vi "DIO-ApplyCorrection.vi"(2 "TaskCluster":T2, 7 "NordSud(ms)":i32, 11 "EstOuest(ms)":i32, 13 "ReferenceCluster":T1) -> (8 "GuiderRA Error":errorcluster, 15 "GuiderDEC Error":errorcluster)   [LabVIEW 2019]
uses:
  <vilib>/DAQmx/write.llb/DAQmx Write (Digital Bool 1Line 1Point).vi
  <vilib>/DAQmx/miscellaneous.llb/DAQmx Fill In Error Info.vi
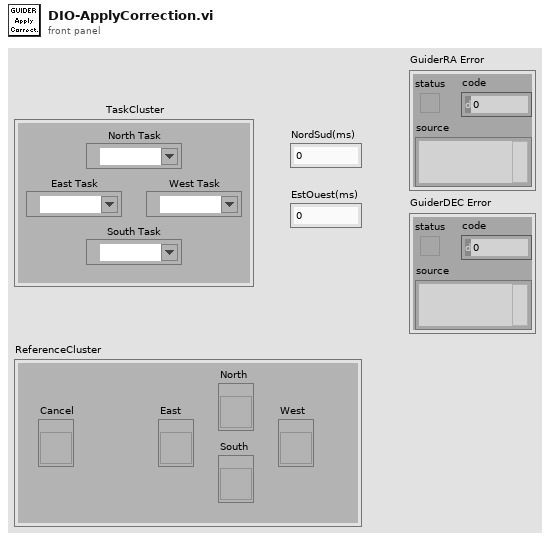
[diagram p1: front panel]
types:
  T1 = cluster{"Cancel":refnum<vi>, "North":refnum<vi>, "South":refnum<vi>, "East":refnum<vi>, "West":refnum<vi>}
  T2 = cluster{"North Task":refnum<k21>, "South Task":refnum<k21>, "East Task":refnum<k21>, "West Task":refnum<k21>}
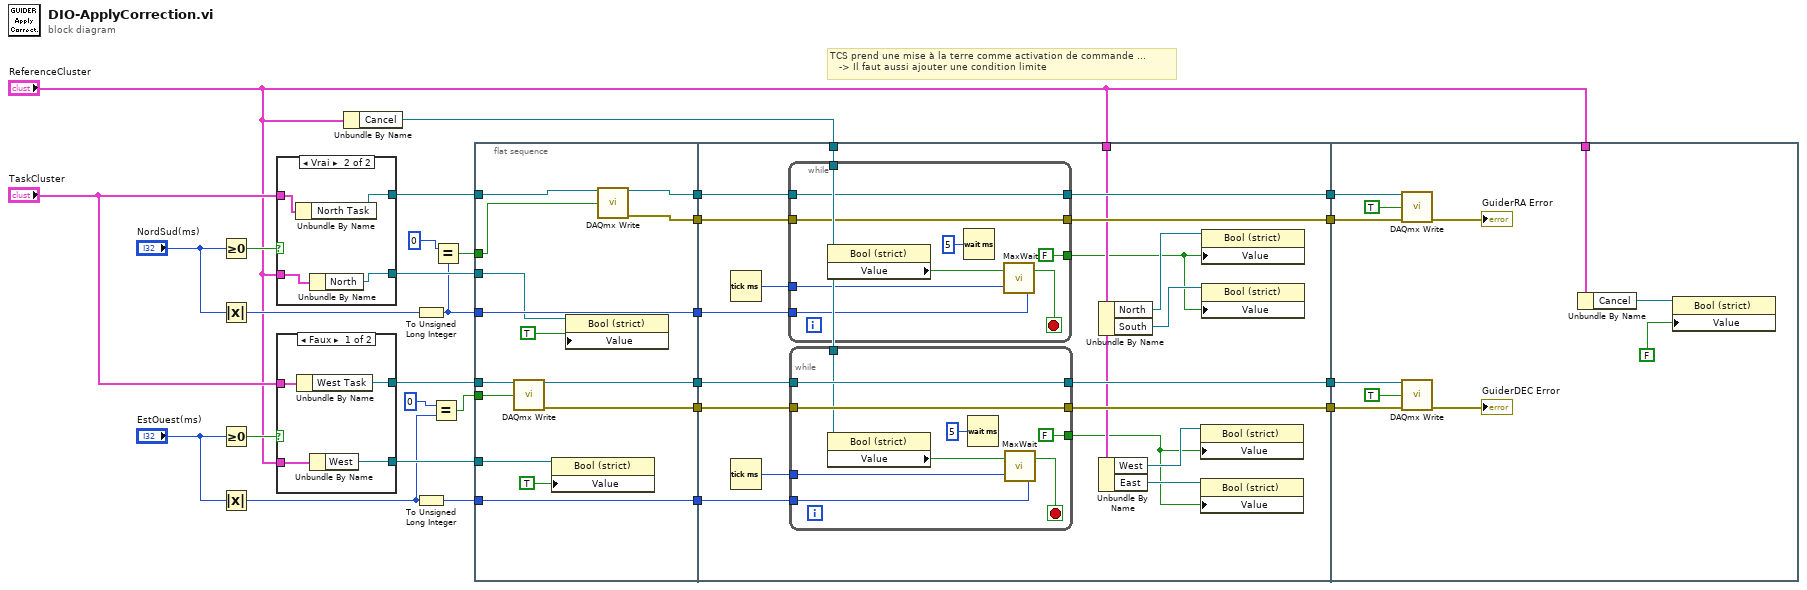
[diagram p0: block diagram]
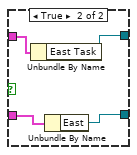
[diagram p2: hidden frame]
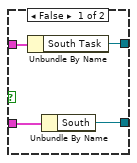
[diagram p3: hidden frame]
diagram:
  # "TCS prend une mise à la terre comme activation de commande ...\n   -> Il faut aussi ajouter une condition limite"
  n1 = Greater Or Equal To 0?(x="NordSud(ms)") -> (x >= 0?=w29:bool)
  n2 = Absolute Value(x="NordSud(ms)") -> (abs(x)=w24:i32)
  n3 = Greater Or Equal To 0?(x="EstOuest(ms)") -> (x >= 0?=w27:bool)
  n4 = Absolute Value(x="EstOuest(ms)") -> (abs(x)=w3:i32)
  n5 = case shown="Vrai" w29 {
    tunnel: "TaskCluster" -> [w33 w37]
    tunnel: [w32 w36] -> w12
    tunnel: "ReferenceCluster" -> [w31 w35]
    tunnel: [w30 w34] -> w15
    frame False {
      n6 = Unbundle By Name(w33) -> ("South Task"=w32:refnum<k21>)
      n7 = Unbundle By Name(w31) -> ("South"=w30:refnum<vi>)
    }
    frame True {
      n8 = Unbundle By Name(w37) -> ("North Task"=w36:refnum<k21>)
      n9 = Unbundle By Name(w35) -> ("North"=w34:refnum<vi>)
    }
  }
  n10 = case shown="Faux" w27 {
    tunnel: "TaskCluster" -> [w41 w45]
    tunnel: [w40 w44] -> w13
    tunnel: "ReferenceCluster" -> [w39 w43]
    tunnel: [w38 w42] -> w14
    frame False {
      n11 = Unbundle By Name(w41) -> ("West Task"=w40:refnum<k21>)
      n12 = Unbundle By Name(w39) -> ("West"=w38:refnum<vi>)
    }
    frame True {
      n13 = Unbundle By Name(w45) -> ("East Task"=w44:refnum<k21>)
      n14 = Unbundle By Name(w43) -> ("East"=w42:refnum<vi>)
    }
  }
  n15 = Unbundle By Name("ReferenceCluster") -> ("Cancel"=w16:refnum<vi>)
  n16 = To Unsigned Long Integer(number=w24) -> (unsigned 32bit integer=w6:u32)
  n17 = To Unsigned Long Integer(number=w3) -> (unsigned 32bit integer=w23:u32)
  n18 = Equal?(x=0, y=w3) -> (x = y?=w1:bool)
  n19 = Equal?(x=u32 0, y=w6) -> (x = y?=w4:bool)
  n20 = flat-sequence {
    tunnel: w23 -> [w58]
    tunnel: w13 -> [w57]
    tunnel: w12 -> [w54]
    tunnel: w6 -> [w59]
    tunnel: [w59] -> w22
    tunnel: [w53] -> w21
    tunnel: [w52] -> w20
    tunnel: [w56] -> w19
    tunnel: [w55] -> w18
    tunnel: [w58] -> w17
    tunnel: w15 -> [w51]
    tunnel: w14 -> [w50]
    tunnel: w4 -> [w47]
    tunnel: w1 -> [w46]
    tunnel: w16 -> [w67]
    tunnel: w22 -> [w79]
    tunnel: w21 -> [w78]
    tunnel: w20 -> [w75]
    tunnel: w19 -> [w73]
    tunnel: w18 -> [w72]
    tunnel: w17 -> [w69]
    tunnel: [w77] -> w11
    tunnel: [w76] -> w10
    tunnel: [w71] -> w9
    tunnel: [w70] -> w8
    tunnel: "ReferenceCluster" -> [w66]
    tunnel: w11 -> [w104]
    tunnel: w10 -> [w103]
    tunnel: w9 -> [w102]
    tunnel: w8 -> [w101]
    tunnel: "ReferenceCluster" -> [w100]
    frame #0 {
      n21 = call-poly <vilib>:"DAQmx Write.vi"("task/channels in"=w57, "data"=w46) -> ("task out"=w56:refnum<k21>, "error out"=w55:errorcluster)  [unwired: 11 in, 1 out]
      n22 = property class="Bool (strict)"(reference=w50, "Value"=TRUE) -> ()  [unwired: 1 in, 2 out]
      n23 = property class="Bool (strict)"(reference=w51, "Value"=TRUE) -> ()  [unwired: 1 in, 2 out]
      n24 = call-poly <vilib>:"DAQmx Write.vi"("task/channels in"=w54, "data"=w47) -> ("task out"=w53:refnum<k21>, "error out"=w52:errorcluster)  [unwired: 11 in, 1 out]
    }
    frame #1 {
      n25 = Tick Count (ms)() -> (millisecond timer value=w74:u32)
      n26 = Tick Count (ms)() -> (millisecond timer value=w68:u32)
      n27 = while {
        tunnel: w79 -> [w94]
        tunnel: w78 -> [w97]
        tunnel: [w97] -> w77
        tunnel: w75 -> [w96]
        tunnel: [w96] -> w76
        tunnel: w74 -> [w95]
        tunnel: w67 -> [w91]
        tunnel: [FALSE] -> w63
        stop <- w93 stop-if-true
        n28 = property class="Bool (strict)"(reference=w91) -> ("Value"=w92:bool)  [unwired: 1 in, 2 out]
        n29 = Wait (ms)(milliseconds to wait=u32 5) -> ()  [unwired: 1 out]
        n30 = call "MaxWait.vi"("WaitLimit (ms)"=w94, "StartTick (from outside the node)"=w95, "Valeur entrante"=w92) -> ("break ?"=w93:bool)
      }
      n31 = while {
        tunnel: w69 -> [w85]
        tunnel: w73 -> [w88]
        tunnel: [w88] -> w71
        tunnel: w72 -> [w87]
        tunnel: [w87] -> w70
        tunnel: w68 -> [w86]
        tunnel: w67 -> [w82]
        tunnel: [FALSE] -> w60
        stop <- w84 stop-if-true
        n32 = property class="Bool (strict)"(reference=w82) -> ("Value"=w83:bool)  [unwired: 1 in, 2 out]
        n33 = Wait (ms)(milliseconds to wait=u32 5) -> ()  [unwired: 1 out]
        n34 = call "MaxWait.vi"("WaitLimit (ms)"=w85, "StartTick (from outside the node)"=w86, "Valeur entrante"=w83) -> ("break ?"=w84:bool)
      }
      n35 = Unbundle By Name(w66) -> ("North"=w65:refnum<vi>, "South"=w64:refnum<vi>)
      n36 = Unbundle By Name(w66) -> ("West"=w61:refnum<vi>, "East"=w62:refnum<vi>)
      n37 = property class="Bool (strict)"(reference=w61, "Value"=w60) -> ()  [unwired: 1 in, 2 out]
      n38 = property class="Bool (strict)"(reference=w62, "Value"=w60) -> ()  [unwired: 1 in, 2 out]
      n39 = property class="Bool (strict)"(reference=w65, "Value"=w63) -> ()  [unwired: 1 in, 2 out]
      n40 = property class="Bool (strict)"(reference=w64, "Value"=w63) -> ()  [unwired: 1 in, 2 out]
    }
    frame #2 {
      n41 = call-poly <vilib>:"DAQmx Write.vi"("task/channels in"=w104, "data"=TRUE, "error in"=w103) -> ("error out"=→"GuiderRA Error":errorcluster)  [unwired: 10 in, 2 out]
      n42 = call-poly <vilib>:"DAQmx Write.vi"("task/channels in"=w102, "data"=TRUE, "error in"=w101) -> ("error out"=→"GuiderDEC Error":errorcluster)  [unwired: 10 in, 2 out]
      n43 = Unbundle By Name(w100) -> ("Cancel"=w99:refnum<vi>)
      n44 = property class="Bool (strict)"(reference=w99, "Value"=FALSE) -> ()  [unwired: 1 in, 2 out]
    }
  }
